vi "Initialize.vi"(7 "Serial Configuration":cluster{"Baud Rate":u32}={"Baud Rate"=9600} {"Baud Rate" items=["38400"=38400, "300"=300, "600"=600, "1200"=1200, "2400"=2400, "4800"=4800, "9600"=9600, "19200"=19200]}, 8 "error in (no error)":errorcluster, 9 "Reset (True)":bool=TRUE, 10 "ID Query (True)":bool=TRUE, 11 "VISA resource name":refnum<visa-resource-name>) -> (0 "error out":errorcluster, 3 "VISA resource name out":refnum<visa-resource-name>)   [LabVIEW 2015, in "IT8900A-E.lvlib"]
doc: "Establishes communication with the instrument and optionally performs an instrument identification query and/or an instrument reset. It also places the instrument in a default state needed for other instrument driver operations. Therefore, call this VI before calling other instrument driver VIs for this instrument. Generally, you need to call the <b>Initialize</b> VI only once at the beginning of an application."
uses:
  <instrlib>/IT8900/IT8900A-E.lvlib
panel:
  # "(c) 2014 <Enter Company Name Here>.  ALL RIGHTS RESERVED."
  # "EDIT: Change control description to remove example text for buses not supported."
  # "EDIT: If your instrument does not support ID query or Reset, remove the ID Query or Reset control from the front panel and delete the case structure with the ID Query or Reset code from the block diagram."
  # "EDIT: Serial settings must match those on the physical instrument.  Review user's manual to determine the correct Flow Control protocol for the instrument.  \"None\" is the least robust option for this setting, and could lead to unreliable data transmission."
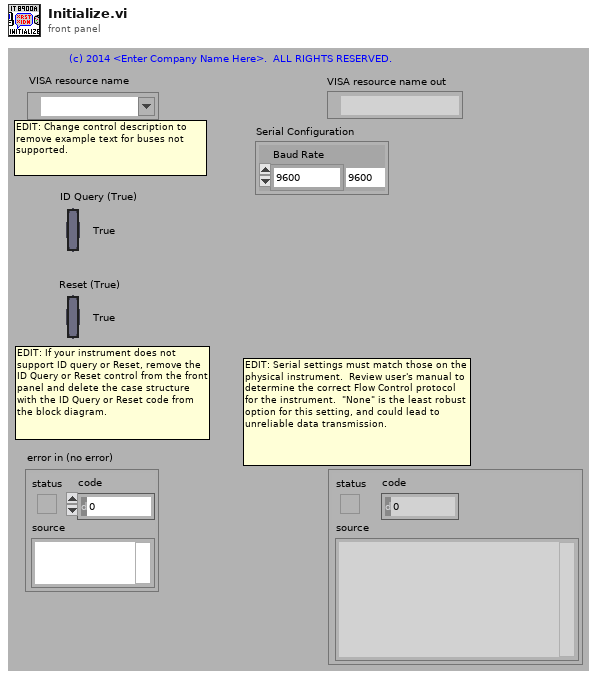
[diagram p1: front panel]
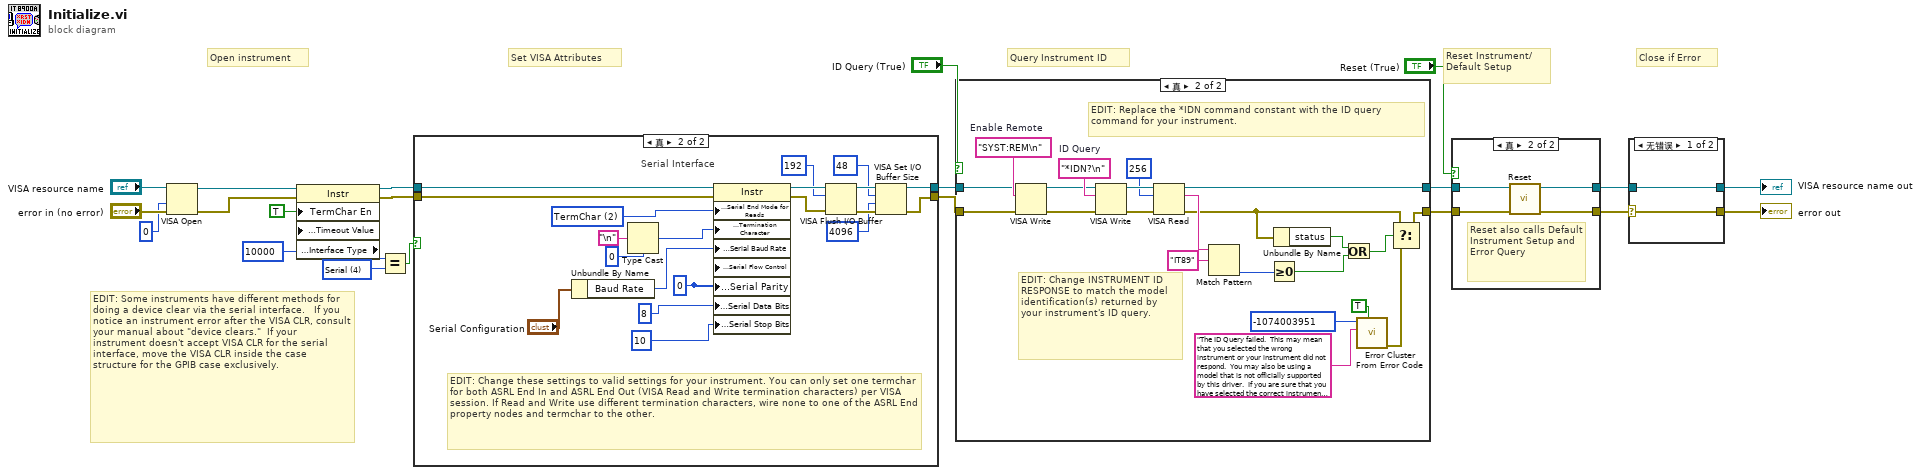
[diagram p0: block diagram]
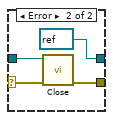
[diagram p3: hidden frame]
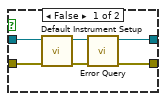
[diagram p4: hidden frame]
diagram:
  w9 = u16 4 items=["GPIB"=1, "VXI"=2, "GPIB-VXI"=3, "Serial"=4, "PXI"=5, "TCPIP"=6, "USB"=7] ("Interface Information:Interface Type")
  # "EDIT: Some instruments have different methods for doing a device clear via the serial interface.   If you notice an instrument error after the VISA CLR, consult your manual about \"device clears.\"  If your instrument doesn't accept VISA CLR for the serial interface, move the VISA CLR inside the case  structure for the GPIB case exclusively."
  # "Set VISA Attributes"
  # "Close if Error"
  # "Query Instrument ID"
  # "Reset Instrument/\nDefault Setup"
  # "Open instrument"
  n1 = VISA Open(access mode=u32 0, error in (no error)="error in (no error)", VISA resource name="VISA resource name") -> (VISA resource name=w3:refnum<visa-resource-name>, error out=w2:errorcluster)  [unwired: 2 in]
  n2 = property class="Instr"(reference=w3, error in=w2, "TermChar En"=TRUE, "General Settings:Timeout Value"=u32 10000) -> (reference out=w12:refnum<visa-resource-name>, error out=w11:errorcluster, "Interface Information:Interface Type"=w16:u16)
  n3 = Equal?(x=w16, y=w9) -> (x = y?=w10:bool)
  n4 = case shown="真" w10 {
    tunnel: [w23 w41] -> w14
    tunnel: [w24 w38] -> w13
    tunnel: w12 -> [w23 w43]
    tunnel: w11 -> [w24 w44]
    frame False {
      # "EDIT: Remove interfaces not supported by your instrument."
      # "GPIB, TCP/IP, and USB Interface"
    }
    frame True {
      w27 = 0
      w31 = u16 2 items=["None", "LastBit", "TermChar"] ("Serial Settings:Serial End Mode for Reads")
      # "EDIT: Change these settings to valid settings for your instrument. You can only set one termchar for both ASRL End In and ASRL End Out (VISA Read and Write termination characters) per VISA session. If Read and Write use different termination characters, wire none to one of the ASRL End property nodes and termchar to the other."
      # "Serial Interface"
      n5 = Unbundle By Name("Serial Configuration") -> ("Baud Rate"=w29:u32)
      n6 = Type Cast(type=u8 0, x="\n" ("Line Feed Constant")) -> (*(type *) &x=w30:u8)
      n7 = property class="Instr"(reference=w43, error in=w44, "Serial Settings:Serial End Mode for Reads"=w31, "Message Based Settings:Termination Character"=w30, "Serial Settings:Serial Baud Rate"=w29, "Serial Settings:Serial Flow Control"=w27, "Serial Settings:Serial Parity"=w27, "Serial Settings:Serial Data Bits"=8, "Serial Settings:Serial Stop Bits"=10) -> (reference out=w37:refnum<visa-resource-name>, error out=w40:errorcluster)
      n8 = VISA Flush I/O Buffer(VISA resource name=w37, mask (16)=u16 192, error in (no error)=w40) -> (VISA resource name out=w42:refnum<visa-resource-name>, error out=w39:errorcluster)
      n9 = VISA Set I/O Buffer Size(VISA resource name=w42, mask (16)=u16 48, size (4096)=u32 4096 ("size (0)"), error in (no error)=w39) -> (VISA resource name out=w41:refnum<visa-resource-name>, error out=w38:errorcluster)
    }
  }
  n10 = case shown="真" "ID Query (True)" {
    tunnel: [w45 w68] -> w21
    tunnel: [w46 w67] -> w22
    tunnel: w14 -> [w46 w48]
    tunnel: w13 -> [w45 w47]
    frame False {
    }
    frame True {
      w51 = "SYST:REM\n"  # Enable Remote
      w61 = "*IDN?\n"  # ID Query
      # "EDIT: Replace the *IDN command constant with the ID query command for your instrument."
      # "EDIT: Change INSTRUMENT ID RESPONSE to match the model identification(s) returned by your instrument's ID query."
      n11 = VISA Write(VISA resource name=w48, write buffer=w51, error in (no error)=w47) -> (VISA resource name out=w50:refnum<visa-resource-name>, error out=w49:errorcluster)  [unwired: 1 out]
      n12 = VISA Write(VISA resource name=w50, write buffer=w61, error in (no error)=w49) -> (VISA resource name out=w65:refnum<visa-resource-name>, error out=w64:errorcluster)  [unwired: 1 out]
      n13 = VISA Read(VISA resource name=w65, byte count=u32 256, error in (no error)=w64) -> (VISA resource name out=w67:refnum<visa-resource-name>, read buffer=w66:string, error out=w55:errorcluster)  [unwired: 1 out]
      n14 = Match Pattern(string=w66, regular expression="IT89") -> (offset past match=w56:i32)  [unwired: 1 in, 3 out]
      n15 = Greater Or Equal To 0?(x=w56) -> (x >= 0?=w53:bool)
      n16 = Unbundle By Name(w55) -> ("status"=w54:bool)
      n17 = Or(x=w54, y=w53) -> (x .or. y?=w52:bool)
      n18 = call <vilib>:"Error Cluster From Error Code.vi"("show call chain? (False)"=TRUE, "error message (\"\")"="The ID Query failed.  This may mean that you selected the wrong instrument or your instrument did not respond.  You may also be using a model that is not officially supported by this driver.  If you are sure that you have selected the correct instrument and it is responding, try disabling the ID Query." ("Source (VI Name)"), "error code (0)"=-1074003951 ("Code")) -> ("error out"=w60:errorcluster)  [unwired: 6 in]
      n19 = Select(t=w55, s=w52, f=w60) -> (s? t:f=w68:errorcluster)
    }
  }
  n20 = case shown="真" "Reset (True)" {
    tunnel: w21 -> [w73 w75]
    tunnel: [w70 w78] -> w4
    tunnel: w22 -> [w74 w76]
    tunnel: [w71 w77] -> w5
    frame False {
      n21 = call <instrlib>:"Default Instrument Setup.vi"("error in (no error)"=w73, "VISA resource name"=w74) -> ("error out"=w69:errorcluster, "VISA resource name out"=w72:refnum<visa-resource-name>)  [unwired: 8 in]
      n22 = call <instrlib>:"Error Query.vi"("error in (no error)"=w69, "VISA resource name"=w72) -> ("error out"=w70:errorcluster, "VISA resource name out"=w71:refnum<visa-resource-name>)  [unwired: 6 in, 2 out]
    }
    frame True {
      # "Reset also calls Default Instrument Setup and Error Query"
      n23 = call <instrlib>:"Reset.vi"("error in (no error)"=w75, "VISA resource name"=w76) -> ("error out"=w78:errorcluster, "VISA resource name out"=w77:refnum<visa-resource-name>)  [unwired: 8 in]
    }
  }
  n24 = case shown="无错误" w4 {
    selector: w4 -> [w79 w82]
    tunnel: w5 -> [w80 w83]
    tunnel: [w80 refnum<visa-resource-name> refnum ("VISA resource name out")] -> w7
    tunnel: [w79 w84] -> w6
    frame No Error {
    }
    frame Error {
      n25 = call <instrlib>:"Close.vi"("error in (no error)"=w82, "VISA resource name"=w83) -> ("error out"=w84:errorcluster)  [unwired: 9 in]
    }
  }
  "VISA resource name out" <- w7
  "error out" <- w6
